vi "test Standard Application Flow.vi"(8 "error in":errorcluster) -> (0 "error out":errorcluster)   [LabVIEW 2020, in "serenial.io-ase.test.lvlib"]
uses:
  serenial.io-ase.test.lvlib
  <vilib>/addons/_JKI Toolkits/Caraya/classes/Assert/Assert.lvclass
  serenial.io-ase/ase/ase.lvclass
  <vilib>/addons/_JKI Toolkits/Caraya/classes/Assert/Assert Not Error.vi
  <vilib>/addons/_JKI Toolkits/Caraya/classes/Assert/Assert Equal Value_Variant.vi
  <vilib>/addons/_JKI Toolkits/Caraya/classes/Test/Test.lvclass
  <vilib>/addons/_JKI Toolkits/Caraya/classes/Assert/Assert Equal Value and Type_Variant.vi
  <vilib>/addons/_JKI Toolkits/Caraya/classes/Assert/Assert True.vi
  serenial.io-ase/ase/Start Call (Exe Path).vi
  Custom ID/Custom ID.lvclass
  C:/serenial/libraries/Asynchronous-System-Executive/LabVIEW/serenial.io-ase/configuration/configuration.lvclass
  C:/serenial/libraries/Asynchronous-System-Executive/LabVIEW/serenial.io-ase.test/Custom ID/Custom ID.lvclass
panel:
  out "Std Err":string
  out "Std Out":string
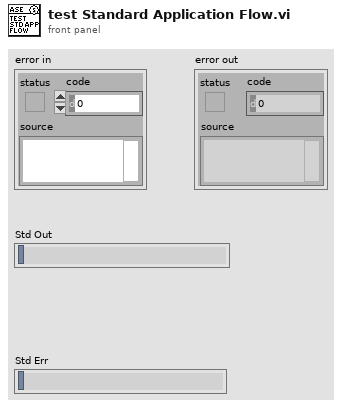
[diagram p1: front panel]
types:
  T1 = typedef "serenial.io-ase.lvlib/ase.lvclass/Event References.ctl" = cluster{"Standard Output":refnum<user-event>, "Standard Error":refnum<user-event>, "Did Exit":refnum<user-event>}
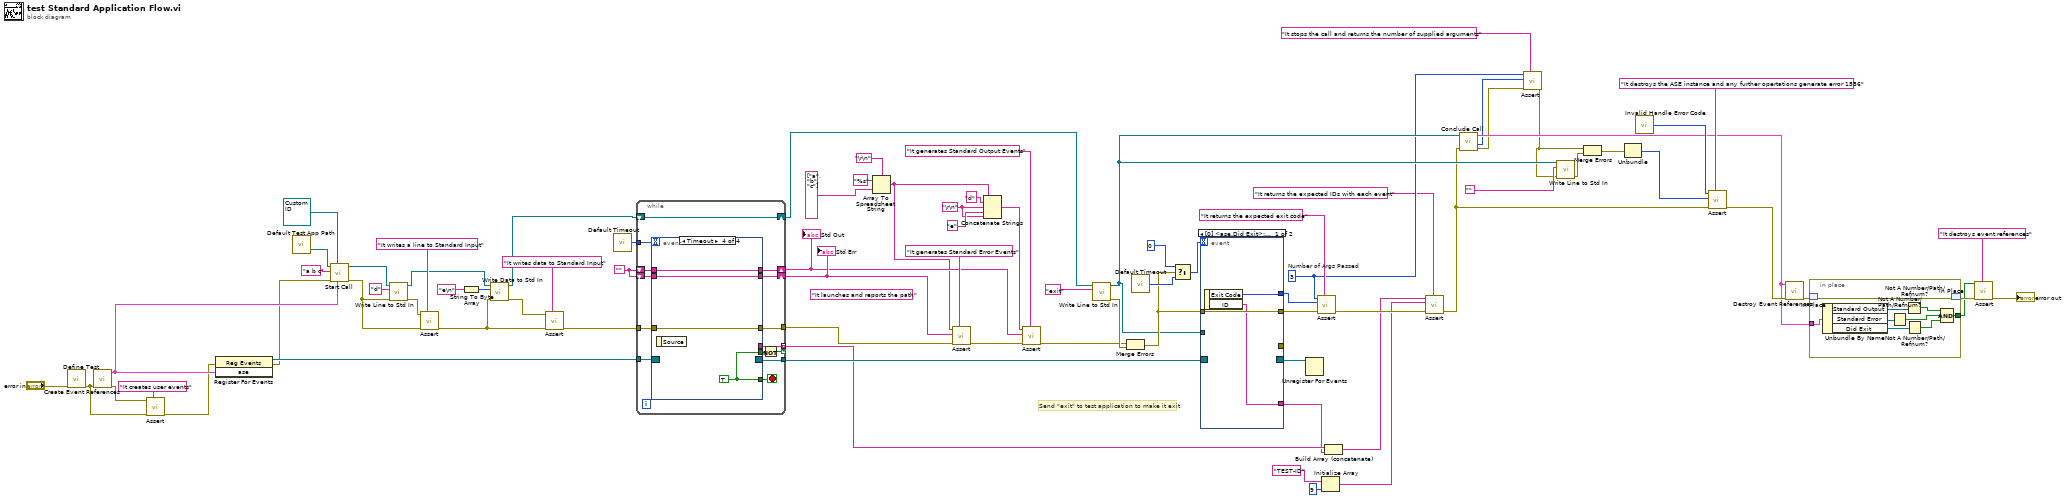
[diagram p0: block diagram]
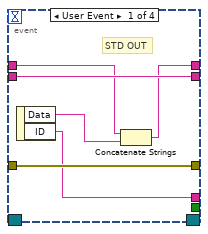
[diagram p2: hidden frame]
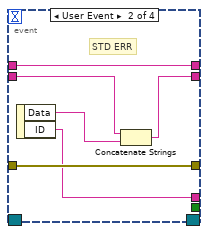
[diagram p3: hidden frame]
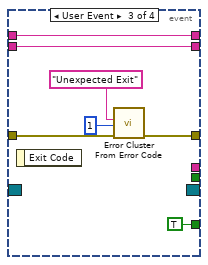
[diagram p4: hidden frame]
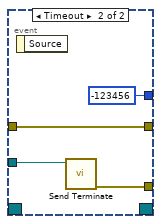
[diagram p5: hidden frame]
diagram:
  w48 = "\r\n"
  w17 = 3  # Number of Args Passed
  w74 = "" ("Empty String Constant")
  (unwired) "It launches and reports the path" ("Label")
  # "Send \"exit\" to test application to make it exit"
  n1 = call <vilib>:"Define Test.vi"("error in (no error)"="error in") -> ("error out"=w41:errorcluster)  [unwired: 10 in]
  n2 = call "Create Event References.vi"("error in"=w41) -> ("error out"=w40:errorcluster, "ase"=w59:T1)  [unwired: 9 in]
  n3 = call-poly <vilib>:"Assert.vi"("Label"="It creates user events", "error in (no error)"=w41, "Not Error?"=w40) -> ("error out"=w39:errorcluster)  [unwired: 8 in]
  n4 = register-events(error in=w39, w59) -> (reference out=w60:refnum<event-registration>, error out=w38:errorcluster)  [unwired: 1 in]
  n5 = call "Default Test App Path.vi"() -> ("Exe Path"=w7:path)  [unwired: 2 in, 1 out]
  n6 = call-poly "Start Call.vi"("Event References"=w59, "Configuration"=refnum<class "Custom ID.lvclass"> refnum ("serenial.io-ase.test.lvlib:Custom ID.lvclass"), "error in"=w38, "Arguments"="a b c", "Executable Path"=w7) -> ("error out"=w47:errorcluster, "New ASE Handle"=w33:refnum<class "ase.lvclass">)  [unwired: 5 in]
  n7 = call "Write Line to Std In .vi"("error in"=w47, "Input"="d", "ASE Handle"=w33) -> ("error out"=w58:errorcluster, "ASE Handle Duplicate"=w31:refnum<class "ase.lvclass">)  [unwired: 6 in, 1 out]
  n8 = call-poly <vilib>:"Assert.vi"("Label"="It writes a line to Standard Input", "error in (no error)"=w47, "Not Error?"=w58) -> ("error out"=w46:errorcluster)  [unwired: 8 in]
  n9 = String To Byte Array(string="e\n") -> (unsigned byte array=w54:u8[])
  n10 = call "Write Data to Std In.vi"("error in"=w46, "Data"=w54, "ASE Handle"=w31) -> ("error out"=w57:errorcluster, "ASE Handle Duplicate"=w25:refnum<class "ase.lvclass">)  [unwired: 6 in, 1 out]
  n11 = call-poly <vilib>:"Assert.vi"("Label"="It writes data to Standard Input", "error in (no error)"=w46, "Not Error?"=w57) -> ("error out"=w80:errorcluster)  [unwired: 8 in]
  n12 = call "Default Timeout.vi"() -> ("Default Timeout"=w73:i32)
  n13 = while {
    tunnel: w80 -> [w95]
    tunnel: w60 -> [w93]
    tunnel: [w92] -> w66
    shift-right: [w87] -> w52
    shift-left: w74 -> [w90]
    shift-right: [w89] -> w72
    shift-left: w74 -> [w88]
    tunnel: w73 -> [w86]
    tunnel: [w94] -> w5
    shift-right: [w85] -> w24
    shift-left: w25 -> [w85]
    tunnel: [w84] -> w16 mode=indexing if=w82
    stop <- w91 stop-if-true
    n14 = event shown="[3] Timeout" {
      selector: w93 -> [_ _ _ _]
      dyn-events: [_ _ _ _] -> w92
      timeout: w86 -> [_ _ _ _]
      tunnel: w95 -> [w101 w107 w110 w118]
      tunnel: [w101 w107 w111 w118] -> w94
      tunnel: [_ _ TRUE w115] -> w91
      tunnel: w90 -> [w98 w105 w114 w116]
      tunnel: [w100 w103 w113 w117] -> w89
      tunnel: w88 -> [w100 w104 w113 w117]
      tunnel: [w97 w105 w114 w116] -> w87
      tunnel: [w96 w102 _ _] -> w84
      tunnel: [_ _ _ w115] -> w83
      event User Event {
        # "STD OUT"
        n15 = event-data() -> ("Data"=w99:string, "ID"=w96:string)  [unwired: 1 in]
        n16 = Concatenate Strings(w98, w99) -> (w97:string)
      }
      event User Event {
        # "STD ERR"
        n17 = event-data() -> ("Data"=w106:string, "ID"=w102:string)  [unwired: 1 in]
        n18 = Concatenate Strings(w104, w106) -> (w103:string)
      }
      event User Event {
        n19 = event-data() -> ()  [unwired: 1 in, 1 out]
        n20 = call <vilib>:"Error Cluster From Error Code.vi"("error in (no error)"=w110, "error message (\"\")"="Unexpected Exit" ("error message (\"\")"), "error code (0)"=1) -> ("error out"=w111:errorcluster)  [unwired: 6 in]
      }
      event Timeout {
        w115 = TRUE
        n21 = event-data() -> ()  [unwired: 1 in, 1 out]
      }
    }
    n22 = Not(x=w83) -> (.not. x?=w82:bool)
  }
  "Std Out" <- w52
  "Std Err" <- w72
  n23 = Array To Spreadsheet String(delimiter (Tab)="\r\n", array=string[] ["a", "b", "c"] ("Arguments"), 3:"%s" ("format string")) -> (spreadsheet string=w6:string)
  n24 = call-poly <vilib>:"Assert.vi"("Label"="It generates Standard Error Events", "error in (no error)"=w5, "Y"=w72, "X"=w6) -> ("error out"=w81:errorcluster)  [unwired: 7 in]
  n25 = Concatenate Strings(w6, "d" ("string"), w48, "e" ("string"), w48) -> (w49:string)
  n26 = call-poly <vilib>:"Assert.vi"("Label"="It generates Standard Output Events", "error in (no error)"=w81, "Y"=w52, "X"=w49) -> ("error out"=w26:errorcluster)  [unwired: 7 in]
  n27 = call "Write Line to Std In .vi"("Input"="exit", "ASE Handle"=w24) -> ("error out"=w45:errorcluster, "ASE Handle Duplicate"=w23:refnum<class "ase.lvclass">)  [unwired: 7 in, 1 out]
  n28 = Merge Errors(w26, w45) -> (w27:errorcluster)
  n29 = call "Default Timeout.vi"() -> ("Default Timeout"=w44:i32)
  n30 = Select(t=0, s=w27, f=w44) -> (s? t:f=w42:i32)
  n31 = event shown="[0] <ase.Did Exit>: User Event" {
    selector: w66 -> [_ _]
    dyn-events: [_ _] -> w65
    timeout: w42 -> [_ _]
    tunnel: w27 -> [w121 w125]
    tunnel: [w121 w125] -> w79
    tunnel: [w120 -123456 ("Exit Code")] -> w63
    tunnel: w23 -> [_ w123]
    tunnel: [_ w122] -> _
    tunnel: [w119 _] -> w15
    event User Event {
      n32 = event-data() -> ("Exit Code"=w120:i32, "ID"=w119:string)  [unwired: 1 in]
    }
    event Timeout {
      n33 = event-data() -> ()  [unwired: 1 in, 1 out]
      n34 = call "Send Terminate.vi"("ASE Handle"=w123) -> ("error out"=w122:errorcluster)  [unwired: 8 in, 2 out]
    }
  }
  n35 = Unregister For Events(event registration refnum=w65) -> ()  [unwired: 1 in, 1 out]
  n36 = call-poly <vilib>:"Assert.vi"("Label"="It returns the expected exit code", "error in (no error)"=w79, "Y"=w63, "X"=w17) -> ("error out"=w14:errorcluster)  [unwired: 7 in]
  n37 = Initialize Array("TEST-ID" ("ID (Default - Empty String)"), 9 ("dimension size")) -> (w8:string[])
  n38 = Build Array (concatenate)(w16, w15) -> (w11:string[])
  n39 = call-poly <vilib>:"Assert.vi"("Label"="It returns the expected IDs with each event", "error in (no error)"=w14, "Y"=w8, "X"=w11) -> ("error out"=w13:errorcluster)  [unwired: 7 in]
  n40 = call "Conclude Call.vi"("error in"=w13, "ASE Handle"=w23) -> ("error out"=w21:errorcluster, "Exit Code"=w19:i32, "Event References"=w22:T1)  [unwired: 7 in]
  n41 = call-poly <vilib>:"Assert.vi"("Label"="It stops the call and returns the number of supplied arguments", "error in (no error)"=w21, "Y"=w19, "X"=w17) -> ("error out"=w20:errorcluster)  [unwired: 7 in]
  n42 = call "Write Line to Std In .vi"("error in"=w20, "Input"="", "ASE Handle"=w23) -> ("error out"=w36:errorcluster)  [unwired: 6 in, 2 out]
  n43 = Merge Errors(w20, w36) -> (w35:errorcluster)
  n44 = Unbundle(w35) -> ("code"=w34:i32)  [unwired: 2 out]
  n45 = call "Invalid Handle Error Code.vi"() -> ("Invalid Handle Error"=w28:i32)
  n46 = call-poly <vilib>:"Assert.vi"("Label"="It destroys the ASE instance and any further opertations generate error 1556", "error in (no error)"=w13, "Y"=w34, "X"=w28) -> ("error out"=w29:errorcluster)  [unwired: 7 in]
  n47 = call "Destroy Event References.vi"("error in"=w29, "Event References"=w22) -> ("error out"=w78:errorcluster)  [unwired: 9 in]
  n48 = in-place "In Place Element Structure" {
    in-place-border: [w130] -> w61
    in-place-border: w22 -> [w126]
    n49 = in-place-match #1 ("In Place In / Out Element")(w78) -> (w134:errorcluster)
    n50 = Unbundle By Name(w126) -> ("Standard Output"=w129:refnum<user-event>, "Standard Error"=w128:refnum<user-event>, "Did Exit"=w127:refnum<user-event>)
    n51 = Not A Number/Path/Refnum?(number/path/refnum=w128) -> (NaN/Path/Refnum?=w132:bool)
    n52 = Not A Number/Path/Refnum?(number/path/refnum=w129) -> (NaN/Path/Refnum?=w133:bool)
    n53 = Not A Number/Path/Refnum?(number/path/refnum=w127) -> (NaN/Path/Refnum?=w131:bool)
    n54 = Compound Arithmetic op=AND(w133, w132, w131) -> (w130:bool)
    n55 = in-place-match #1 ("In Place In / Out Element")(w134) -> (w77:errorcluster)
  }
  n56 = call-poly <vilib>:"Assert.vi"("Label"="It destroys event references", "error in (no error)"=w77, "True?"=w61) -> ("error out"=→"error out":errorcluster)  [unwired: 8 in]
